vi "LLM_Spctrm_Params.vi"(0 "Data":dbl[][](array[numeric])=array6401x2[12802 elements]) -> (1 "Pmax / dBm":dbl, 2 "Pmax / nW":dbl, 3 "Fmax / MHz":dbl, 4 "LL / MHz":dbl)   [LabVIEW 2020]
doc: "Determine peak value of spectrum and its frequency location\n\nR. Sheehan 26 - 10 - 2021"
uses:
  Equal With Epsilon Functor.lvclass
  Equal With Epsilon Functor.lvclass/Equal With Epsilon Functor.ctl
  c590df87-7917-4d9b-931c-d88a61146daf.vi
  c590df87-7917-4d9b-931c-d88a61146daf.vi/5f008cf9-0835-42d5-ab12-715ade7a221f.vi
  c590df87-7917-4d9b-931c-d88a61146daf.vi/5f008cf9-0835-42d5-ab12-715ade7a221f.vi/4a937600-749b-4ff4-8f55-34e6a7c3203b.vi
  Equals.vi
panel:
  out "PHM / dBm":dbl
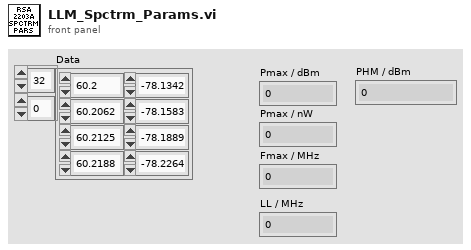
[diagram p1: front panel]
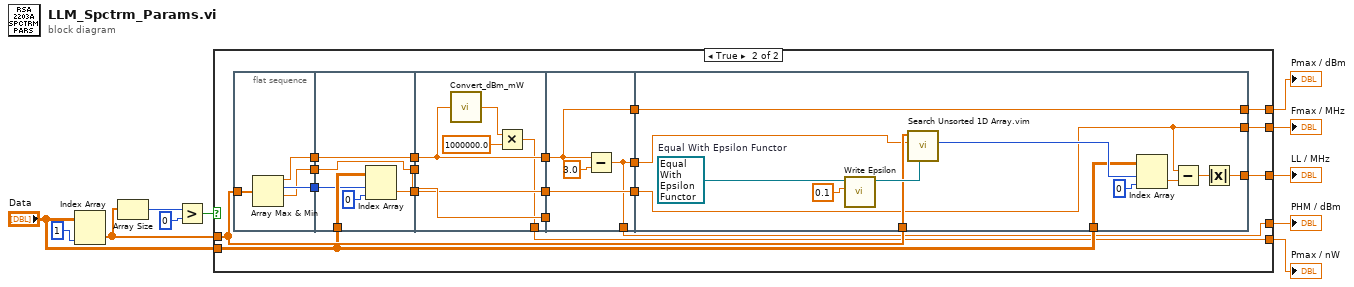
[diagram p0: block diagram]
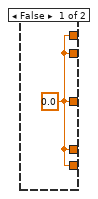
[diagram p2: hidden frame]
diagram:
  n1 = Index Array(array="Data", index (col)=1 ("disabled index (col)")) -> (element=w6:dbl[])  [unwired: 1 in]
  n2 = Array Size(array=w6) -> (size(s)=w11:i32)
  n3 = Greater?(x=w11, y=0) -> (0:w9:bool)
  n4 = case shown="True" w9 {
    tunnel: w6 -> [_ w22]
    tunnel: [w12 w13] -> w4
    tunnel: [w12 w31] -> w8
    tunnel: "Data" -> [_ w21]
    tunnel: [w12 w16] -> w5
    tunnel: [w12 w17] -> w3
    tunnel: [w12 w14] -> w1
    frame False {
      w12 = 0.0
    }
    frame True {
      n5 = flat-sequence {
        tunnel: w22 -> [w34]
        tunnel: [w35] -> w30
        tunnel: [w33] -> w29
        tunnel: [w32] -> w28
        tunnel: w30 -> [w38]
        tunnel: w29 -> [w41]
        tunnel: w28 -> [w40]
        tunnel: w21 -> [w39]
        tunnel: [w41] -> w27
        tunnel: [w40] -> w26
        tunnel: [w36] -> w18
        tunnel: w27 -> [w47]
        tunnel: w26 -> [w46]
        tunnel: [w47] -> w25
        tunnel: [w46] -> w24
        tunnel: [w45] -> w19
        tunnel: w18 -> [w45]
        tunnel: [w42] -> w13
        tunnel: w25 -> [_]
        tunnel: w24 -> [w50]
        tunnel: [w50] -> w23
        tunnel: [w51] -> w20
        tunnel: w19 -> [w51]
        tunnel: [w48] -> w15
        tunnel: [w48] -> w14
        tunnel: w23 -> [w64]
        tunnel: w22 -> [w60]
        tunnel: w21 -> [w58]
        tunnel: [w64] -> w31
        tunnel: w20 -> [w53]
        tunnel: [w54] -> w17
        tunnel: [w53] -> w16
        tunnel: w15 -> [w52]
        frame #0 {
          n6 = Array Max & Min(array=w34) -> (max value=w32:dbl, max index (indices)=w35:i32, min value=w33:dbl)  [unwired: 1 out]
        }
        frame #1 {
          n7 = Index Array(array=w39, index (row)=w38, index (col)=0 ("disabled index (col)")) -> (element=w36:dbl)
        }
        frame #2 {
          n8 = call "Convert_dBm_mW.vi"("Power (dBm)"=w46) -> ("Power (mW)"=w44:dbl)
          n9 = Multiply(x=w44, y=1000000.0) -> (x*y=w42:dbl)
        }
        frame #3 {
          n10 = Subtract(x=w50, y=3.0) -> (x-y=w48:dbl)
        }
        frame #4 {
          w61 = refnum<class "Equal With Epsilon Functor.lvclass"> refnum  # Equal With Epsilon Functor
          n11 = call "Write Epsilon.vi"("epsilon"=0.1, "Equal With Epsilon Functor in"=w61) -> ("Equal With Epsilon Functor out"=w63:refnum<class "Equal With Epsilon Functor.lvclass">)  [unwired: 9 in]
          n12 = call "Search Unsorted 1D Array.vim"("equals function (built-in =)"=w63, "element"=w52, "unsorted 1D array"=w60) -> ("index of element"=w59:i32)  [unwired: 8 in]
          n13 = Index Array(array=w58, index (row)=w59, index (col)=0 ("disabled index (col)")) -> (element=w56:dbl)
          n14 = Subtract(x=w53, y=w56) -> (x-y=w55:dbl)
          n15 = Absolute Value(x=w55) -> (abs(x)=w54:dbl)
        }
      }
    }
  }
  "LL / MHz" <- w3
  "Pmax / dBm" <- w8
  "Fmax / MHz" <- w5
  "Pmax / nW" <- w4
  "PHM / dBm" <- w1
